vi "AdjustSettings.vi"(9 "Smoothing":i32, 10 "Averaging":i32=1, 11 "Integration Time (msec)":i32=10) -> (3 "Spectrometer Settings":T1(array[cluster]))   [LabVIEW 2012]
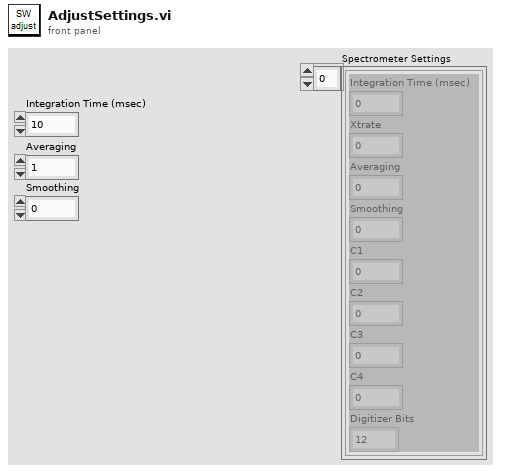
[diagram p1: front panel]
types:
  T1 = cluster{"Integration Time (msec)":i32, "Xtrate":i32, "Averaging":i32, "Smoothing":i32, "C1":dbl, "C2":dbl, "C3":dbl, "C4":dbl, "Digitizer Bits":enum8{"12", "14", "16"}}[]
  T2 = cluster{"Integration Time (msec)":i32, "Xtrate":i32, "Averaging":i32, "Smoothing":i32, "C1":dbl, "C2":dbl, "C3":dbl, "C4":dbl, "Digitizer Bits":enum8{"12", "14", "16"}}
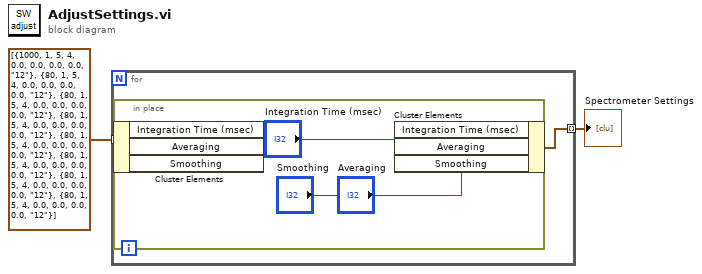
[diagram p0: block diagram]
diagram:
  n1 = for {
    tunnel: T1 [{"Integration Time (msec)"=1000, "Xtrate"=1, "Averaging"=5, "Smoothing"=4, "C1"=0.0, "C2"=0.0, "C3"=0.0, "C4"=0.0, "Digitizer Bits"=enum."12"}, {"Integration Time (msec)"=80, "Xtrate"=1, "Averaging"=5, "Smoothing"=4, "C1"=0.0, "C2"=0.0, "C3"=0.0, "C4"=0.0, "Digitizer Bits"=enum."12"}, {"Integration Time (msec)"=80, "Xtrate"=1, "Averaging"=5, "Smoothing"=4, "C1"=0.0, "C2"=0.0, "C3"=0.0, "C4"=0.0, "Digitizer Bits"=enum."12"}, {"Integration Time (msec)"=80, "Xtrate"=1, "Averaging"=5, "Smoothing"=4, "C1"=0.0, "C2"=0.0, "C3"=0.0, "C4"=0.0, "Digitizer Bits"=enum."12"}, {"Integration Time (msec)"=80, "Xtrate"=1, "Averaging"=5, "Smoothing"=4, "C1"=0.0, "C2"=0.0, "C3"=0.0, "C4"=0.0, "Digitizer Bits"=enum."12"}, {"Integration Time (msec)"=80, "Xtrate"=1, "Averaging"=5, "Smoothing"=4, "C1"=0.0, "C2"=0.0, "C3"=0.0, "C4"=0.0, "Digitizer Bits"=enum."12"}, {"Integration Time (msec)"=80, "Xtrate"=1, "Averaging"=5, "Smoothing"=4, "C1"=0.0, "C2"=0.0, "C3"=0.0, "C4"=0.0, "Digitizer Bits"=enum."12"}, {"Integration Time (msec)"=80, "Xtrate"=1, "Averaging"=5, "Smoothing"=4, "C1"=0.0, "C2"=0.0, "C3"=0.0, "C4"=0.0, "Digitizer Bits"=enum."12"}] ("Channel Settings") -> [w4] mode=indexing
    tunnel: [w3] -> w1 mode=indexing
    n2 = in-place {
      n3 = in-place-cluster #1(w4) -> ()  [unwired: 3 out]
      n4 = in-place-cluster #1("Integration Time (msec)"="Integration Time (msec)", "Averaging"="Averaging", "Smoothing"="Smoothing") -> (w3:T2)
    }
  }
  "Spectrometer Settings" <- w1
